vi "Send Pulse.vi"(8 "error in (no error)":errorcluster, 11 "Sync Box in":refnum<class "Sync Box.lvclass">) -> (0 "error out":errorcluster, 1 "Init acquisition time":dbl format="%.2f", 3 "Sync Box out":refnum<class "Sync Box.lvclass">)   [LabVIEW 2018, in "Sync Box.lvclass"]
uses:
  Sync Box.lvclass
  Sync Box.lvclass/Sync Box.ctl
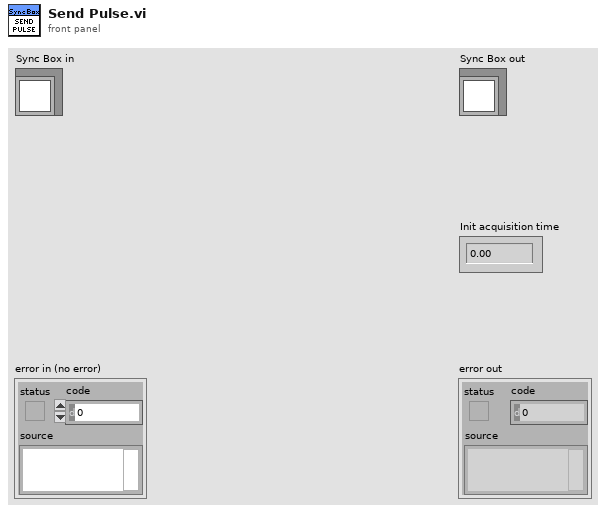
[diagram p1: front panel]
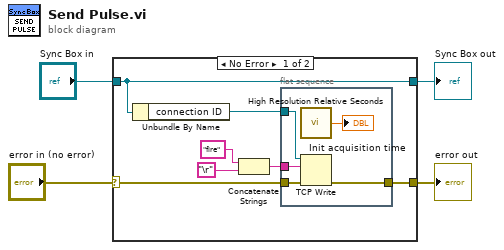
[diagram p0: block diagram]
diagram:
  n1 = case shown="No Error" "error in (no error)" {
    selector: "error in (no error)" -> [w11 w18]
    tunnel: [w10 w18] -> w3
    tunnel: [w5 w17] -> w1
    tunnel: "Sync Box in" -> [w5 w17]
    frame No Error {
      n2 = Unbundle By Name(w5) -> ("connection ID"=w9:refnum<k5>)
      n3 = Concatenate Strings("fire", "\r") -> (w8:string)
      n4 = flat-sequence {
        tunnel: w11 -> [w16]
        tunnel: [w15] -> w10
        tunnel: w9 -> [w14]
        tunnel: w8 -> [w13]
        frame #0 {
          n5 = call <vilib>:"High Resolution Relative Seconds.vi"() -> ("relative seconds"=→"Init acquisition time":dbl)
          n6 = TCP Write(connection ID=w14, data in=w13, error in (no error)=w16) -> (error out=w15:errorcluster)  [unwired: 1 in, 2 out]
        }
      }
    }
    frame Error {
    }
  }
  "error out" <- w3
  "Sync Box out" <- w1
